vi "Odour_valve_waveforms.vi"(1 "Pre-sampling (ms)":dbl format="%#_13g", 2 "Stim parameters":T1={"Name"="", "VPs"=[], "Concentrations (ppm)"=[], "Back valve ON delays"=[], "Back valve OFF delays"=[], "Pulse duration (ms)"=250.0, "Step duration (ms)"=2.0, "Sampling rate (Hz)"=20000.0}) -> (0 "Digital waveform array":digitalwaveform[](array[waveform]))   [LabVIEW 2016]
uses:
  <vilib>/Waveform/DWDTOps.llb/DWDT Boolean Array to Digital.vi
panel:
  out "size(s)":i32[](array[numeric])
  in  "index":i32=6
  in  "TTL binary step duration (ms)":dbl format="%#_13g"
  out "digital waveform":digitalwaveform(graph)
  out "appended array":bool[](array[boolean])
  out "element":digitalwaveform(graph)
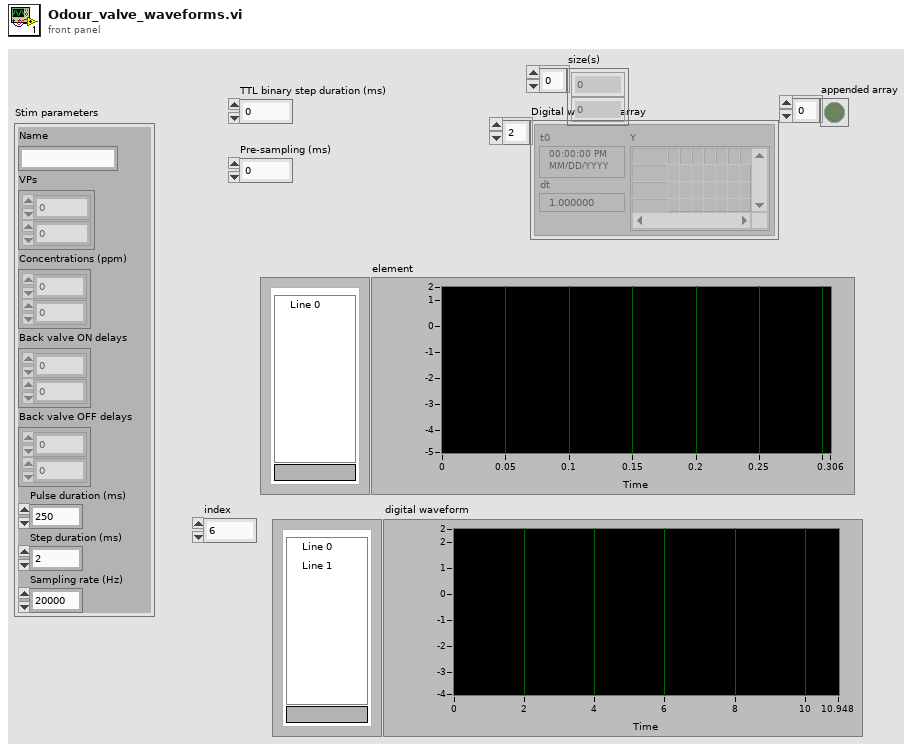
[diagram p1: front panel]
types:
  T1 = cluster{"Name":string, "VPs":dbl[], "Concentrations (ppm)":dbl[], "Back valve ON delays":dbl[], "Back valve OFF delays":dbl[], "Pulse duration (ms)":dbl, "Step duration (ms)":dbl, "Sampling rate (Hz)":dbl}
  T2 = cluster{"Conc. (ppm)":dbl, "Pulse duration (ms)":dbl, "Step duration (ms)":dbl, "Sampling rate (Hz)":dbl, "Back valve ON delay (ms)":dbl, "Back valve OFF delay (ms)":dbl, "VP (Hgmm)":dbl}
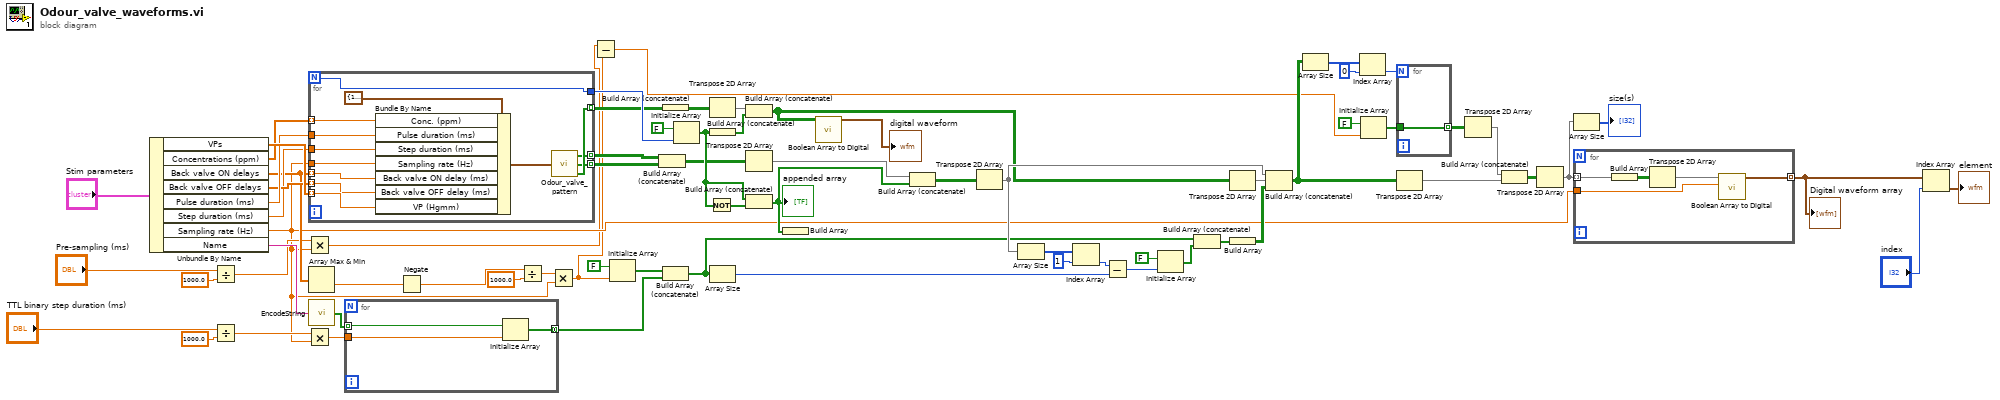
[diagram p0: block diagram]
diagram:
  n1 = Unbundle By Name("Stim parameters") -> ("VPs"=w66:dbl[], "Concentrations (ppm)"=w65:dbl[], "Back valve ON delays"=w28:dbl[], "Back valve OFF delays"=w63:dbl[], "Pulse duration (ms)"=w64:dbl, "Step duration (ms)"=w47:dbl, "Sampling rate (Hz)"=w16:dbl, "Name"=w58:string)
  n2 = Divide(x="Pre-sampling (ms)", y=1000.0) -> (x/y=w17:dbl)
  n3 = Divide(x="TTL binary step duration (ms)", y=1000.0) -> (x/y=w33:dbl)
  n4 = Multiply(x=w17, y=w16) -> (x*y=w15:dbl)
  n5 = Multiply(x=w33, y=w16) -> (x*y=w31:dbl)
  n6 = for {
    N -> [w81]
    tunnel: [w72] -> w57 mode=indexing
    tunnel: [w71] -> w46 mode=indexing
    tunnel: [w73] -> w40 mode=indexing
    tunnel: [w81] -> w70
    tunnel: w66 -> [w80] mode=indexing
    tunnel: w65 -> [w79] mode=indexing
    tunnel: w64 -> [w78]
    tunnel: w47 -> [w77]
    tunnel: w16 -> [w76]
    tunnel: w28 -> [w75] mode=indexing
    tunnel: w63 -> [w74] mode=indexing
    n7 = Bundle By Name(cluster=T2 {"Conc. (ppm)"=10.0, "Pulse duration (ms)"=250.0, "Step duration (ms)"=2.0, "Sampling rate (Hz)"=20000.0, "Back valve ON delay (ms)"=-50.0, "Back valve OFF delay (ms)"=50.0, "VP (Hgmm)"=1.0} ("Pulse parameters"), "Conc. (ppm)"=w79, "Pulse duration (ms)"=w78, "Step duration (ms)"=w77, "Sampling rate (Hz)"=w76, "Back valve ON delay (ms)"=w75, "Back valve OFF delay (ms)"=w74, "VP (Hgmm)"=w80) -> (w82:T2)
    n8 = call "Odour_valve_pattern.vi"("Pulse parameters"=w82) -> ("back valve pattern"=w73:bool[], "counter valve pattern"=w71:bool[], "odour valve pattern"=w72:bool[])  [unwired: 2 in]
  }
  n9 = Array Max & Min(array=w28) -> (min value=w27:dbl)  [unwired: 3 out]
  n10 = call "EncodeString.vi"("string"=w58) -> ("Boolean array"=w32:bool[])
  n11 = for {
    tunnel: w32 -> [w86] mode=indexing
    tunnel: w31 -> [w85]
    tunnel: [w84] -> w21 mode=concatenating
    n12 = Initialize Array(w86, w85) -> (w84:bool[])
  }
  n13 = Negate(x=w27) -> (-x=w25:dbl)
  n14 = Divide(x=w25, y=1000.0) -> (x/y=w24:dbl)
  n15 = Multiply(x=w24, y=w16) -> (x*y=w14:dbl)
  n16 = Subtract(x=w15, y=w14) -> (x-y=w12:dbl)
  n17 = Initialize Array(FALSE, w14) -> (w22:bool[])
  n18 = Build Array (concatenate)(w57, w46) -> (w56:bool[][])
  n19 = Build Array (concatenate)(w40) -> (w62:bool[][])
  n20 = Build Array (concatenate)(w22, w21) -> (w20:bool[])
  n21 = Initialize Array(FALSE, w70) -> (w59:bool[])
  n22 = Not(x=w59) -> (.not. x?=w68:bool[])
  n23 = Transpose 2D Array(2D array=w62) -> (transposed array=w61:bool[][])
  n24 = Build Array (concatenate)(w59) -> (w60:bool[])
  n25 = Array Size(array=w20) -> (size(s)=w52:i32)
  n26 = Build Array (concatenate)(w61, w60) -> (w29:bool[][])
  n27 = Transpose 2D Array(2D array=w56) -> (transposed array=w44:bool[][])
  n28 = Build Array (concatenate)(w59, w68) -> (w39:bool[])
  "appended array" <- w39
  n29 = Build Array(w39) -> ()  [unwired: 1 out]
  n30 = call-poly <vilib>:"Boolean Array to Digital.vi"("boolean array"=w29) -> ("digital waveform"=→"digital waveform":digitalwaveform)  [unwired: 9 in, 1 out]
  n31 = Build Array (concatenate)(w44, w39) -> (w36:bool[][])
  n32 = Transpose 2D Array(2D array=w36) -> (transposed array=w37:bool[][])
  n33 = Array Size(array=w37) -> (size(s)=w55:i32[])
  n34 = Index Array(array=w55, index=1) -> (element=w53:i32)
  n35 = Subtract(x=w53, y=w52) -> (x-y=w50:i32)
  n36 = Initialize Array(FALSE ("element"), w50) -> (w49:bool[])
  n37 = Build Array (concatenate)(w20, w49) -> (w45:bool[])
  n38 = Transpose 2D Array(2D array=w29) -> (transposed array=w30:bool[][])
  n39 = Build Array(w45) -> (w48:bool[][])
  n40 = Build Array (concatenate)(w37, w30, w48) -> (w13:bool[][])
  n41 = Array Size(array=w13) -> (size(s)=w9:i32[])
  n42 = Index Array(array=w9, index=0) -> (element=w7:i32)
  n43 = Initialize Array(FALSE, w12) -> (w10:bool[])
  n44 = for {
    N: w7 -> [_]
    tunnel: [w87] -> w6 mode=indexing
    tunnel: w10 -> [w87]
  }
  n45 = Transpose 2D Array(2D array=w13) -> (transposed array=w2:bool[][])
  n46 = Transpose 2D Array(2D array=w6) -> (transposed array=w3:bool[][])
  n47 = Build Array (concatenate)(w3, w2) -> (w5:bool[][])
  n48 = Transpose 2D Array(2D array=w5) -> (transposed array=w1:bool[][])
  n49 = Array Size(array=w1) -> (size(s)=→"size(s)":i32[])
  n50 = for {
    tunnel: w1 -> [w91] mode=indexing
    tunnel: [w92] -> w43 mode=indexing
    tunnel: w16 -> [w88]
    n51 = Build Array(w91) -> (w90:bool[][])
    n52 = Transpose 2D Array(2D array=w90) -> (transposed array=w89:bool[][])
    n53 = call-poly <vilib>:"Boolean Array to Digital.vi"("sample rate"=w88, "boolean array"=w89) -> ("digital waveform"=w92:digitalwaveform)  [unwired: 8 in, 1 out]
  }
  "Digital waveform array" <- w43
  n54 = Index Array(array=w43, index="index") -> (element=→"element":digitalwaveform)
